vi "Write Timing.vi"(8 "error in (no error)":errorcluster, 10 "Time":dbl, 11 "Sim Display Console Actor in":refnum<class "Sim Display Console Actor.lvclass">) -> (0 "error out":errorcluster, 3 "Sim Display Console Actor out":refnum<class "Sim Display Console Actor.lvclass">)   [LabVIEW 2019, in "Simulated Display Console Actor.lvlib" / "Sim Display Console Actor.lvclass"]
uses:
  Sim Display Console Actor.lvclass
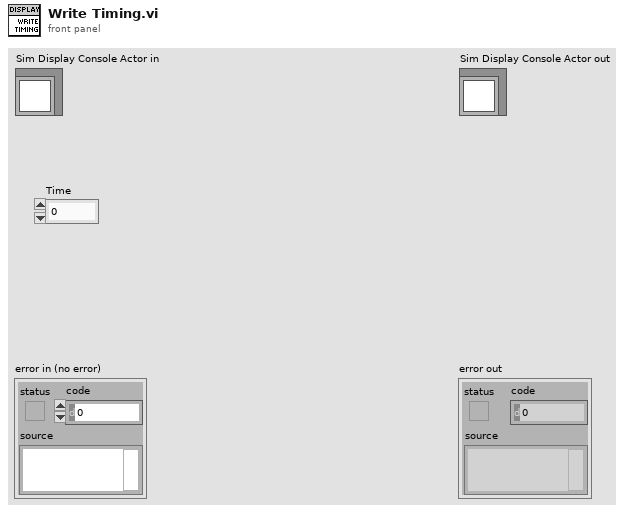
[diagram p1: front panel]
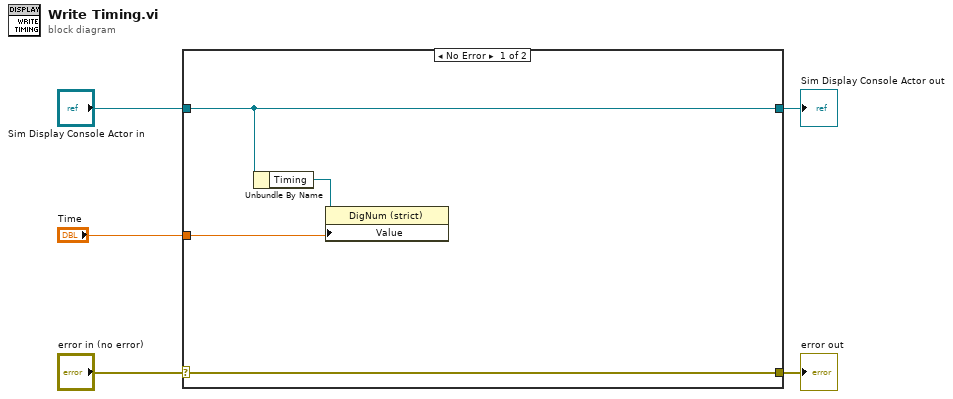
[diagram p0: block diagram]
diagram:
  n1 = case shown="No Error" "error in (no error)" {
    selector: "error in (no error)" -> [w9 w11]
    tunnel: [w9 w11] -> w4
    tunnel: [w8 w10] -> w2
    tunnel: "Sim Display Console Actor in" -> [w8 w10]
    tunnel: "Time" -> [w6 _]
    frame No Error {
      n2 = Unbundle By Name(w8) -> ("Timing"=w7:refnum<vi>)
      n3 = property class="DigNum (strict)"(reference=w7, "Value"=w6) -> ()  [unwired: 1 in, 2 out]
    }
    frame Error {
    }
  }
  "error out" <- w4
  "Sim Display Console Actor out" <- w2
